vi "Center2.vi"(8 "error in (no error)":errorcluster, 9 "Width":dbl=420.0 format="%#_13g", 10 "Height":dbl=560.0 format="%#_13g", 11 "VI in":refnum<vi>) -> (0 "error out":errorcluster, 1 "New Bounds":T1, 2 "Active Monitor":u16)   [LabVIEW 2018]
uses:
  <vilib>/Utility/miscctls.llb/LVRectTypeDef.ctl
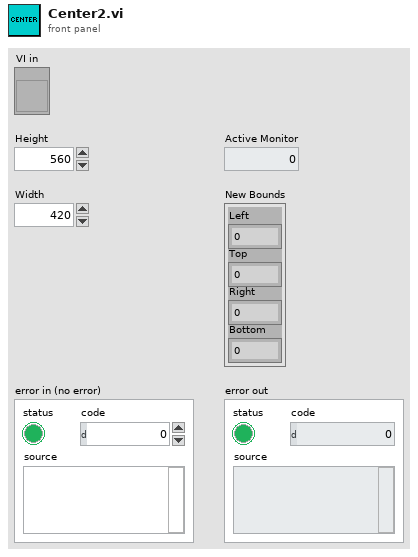
[diagram p1: front panel]
types:
  T1 = typedef "LVRectTypeDef.ctl" = cluster{"Left":i16, "Top":i16, "Right":i16, "Bottom":i16}
  T2 = cluster{"Left":dbl, "Top":dbl, "Right":dbl, "Bottom":dbl}
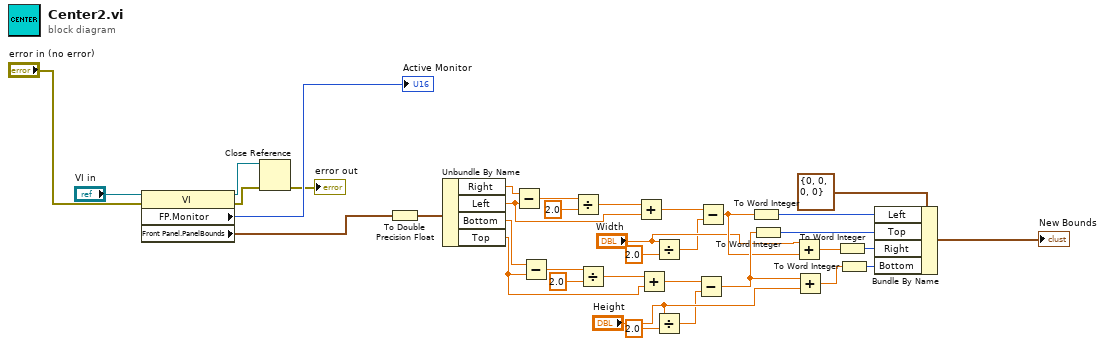
[diagram p0: block diagram]
diagram:
  n1 = property class="VI"(reference="VI in", error in="error in (no error)") -> (reference out=w2:refnum<vi>, error out=w3:errorcluster, "FP.Monitor"=→"Active Monitor":u16, "Front Panel.PanelBounds"=w10:T1)
  n2 = Close Reference(reference=w2, error in (no error)=w3) -> (error out=→"error out":errorcluster)
  n3 = To Double Precision Float(number=w10) -> (double precision float=w11:T2)
  n4 = Unbundle By Name(w11) -> ("Right"=w20:dbl, "Left"=w14:dbl, "Bottom"=w6:dbl, "Top"=w18:dbl)
  n5 = Subtract(x=w20, y=w14) -> (x-y=w7:dbl)
  n6 = Subtract(x=w6, y=w18) -> (x-y=w8:dbl)
  n7 = Divide(x=w7, y=2.0) -> (x/y=w9:dbl)
  n8 = Divide(x=w8, y=2.0) -> (x/y=w17:dbl)
  n9 = Add(x=w9, y=w14) -> (x+y=w19:dbl)
  n10 = Add(x=w17, y=w18) -> (x+y=w30:dbl)
  n11 = Divide(x="Width", y=2.0) -> (x/y=w28:dbl)
  n12 = Divide(x="Height", y=2.0) -> (x/y=w22:dbl)
  n13 = Subtract(x=w30, y=w22) -> (x-y=w35:dbl)
  n14 = Subtract(x=w19, y=w28) -> (x-y=w34:dbl)
  n15 = To Word Integer(number=w34) -> (16bit integer=w21:i16)
  n16 = To Word Integer(number=w35) -> (16bit integer=w23:i16)
  n17 = Add(x="Width", y=w34) -> (x+y=w27:dbl)
  n18 = Add(x=w35, y="Height") -> (x+y=w26:dbl)
  n19 = To Word Integer(number=w27) -> (16bit integer=w24:i16)
  n20 = To Word Integer(number=w26) -> (16bit integer=w25:i16)
  n21 = Bundle By Name(cluster=T1 {"Left"=0, "Top"=0, "Right"=0, "Bottom"=0} ("Front Panel Window:Panel Bounds"), "Left"=w21, "Top"=w23, "Right"=w24, "Bottom"=w25) -> (→"New Bounds":T1)
